vi "CREATE VECTOR FROM SELECTION.vi"(0 "RadioButtonsControl in":refnum<vi>, 1 "Ts (Sampling Rate)":u16(ring) items=["1000 sec"=0, "100 msec"=8, "10 msec"=4, "1 msec"=2, "100 usec"=1], 2 "Digital (pin2) conf":enum32{"Item 0", "Item 1"}(radio), 3 "A3":bool, 4 "Digital (pin4) conf":enum32{"Item 0", "Item 1"}(radio), 6 "RadioBtnsControl Refnum in":refnum<vi>, 7 "enable DIO":bool, 8 "A0":bool, 9 "A5":bool, 10 "A1":bool, 11 "A2":bool, 13 "A4":bool) -> (15 "Array":bool[](array[boolean]))   [LabVIEW 2018]
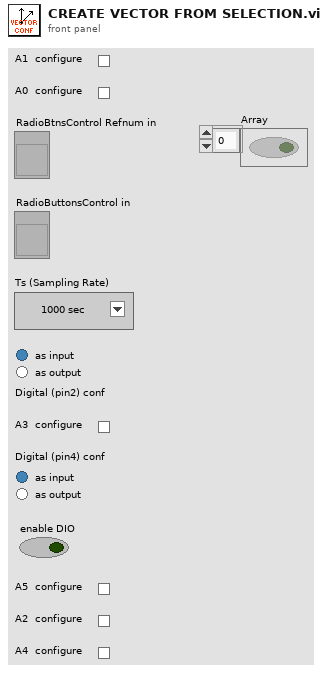
[diagram p1: front panel]
types:
  T1 = enum8{"Enabled", "Disabled", "Disabled and Grayed Out"}
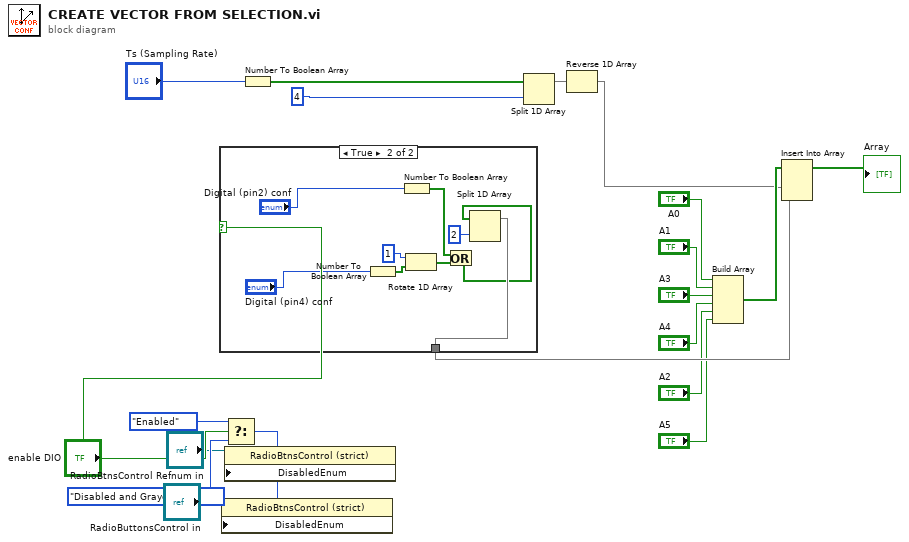
[diagram p0: block diagram]
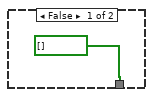
[diagram p2: hidden frame]
diagram:
  n1 = case shown="True" "enable DIO" {
    tunnel: [bool[] [] ("x .or. y?") w24] -> w19
    frame False {
    }
    frame True {
      n2 = Number To Boolean Array(number="Digital (pin4) conf") -> (Boolean array=w28:bool[])
      n3 = Number To Boolean Array(number="Digital (pin2) conf") -> (Boolean array=w29:bool[])
      n4 = Rotate 1D Array(1:w28, 2:1 ("n")) -> (0:w27:bool[])
      n5 = Or(x=w29, y=w27) -> (x .or. y?=w23:bool[])
      n6 = Split 1D Array(array=w23, index=2) -> (first subarray=w24:bool[])  [unwired: 1 out]
    }
  }
  n7 = Select(t=T1."Enabled" ("Disabled"), s="enable DIO", f=T1."Disabled and Grayed Out" ("Disabled")) -> (s? t:f=w16:T1)
  n8 = property on="Property Node" class="RadioBtnsControl (strict)"(reference="RadioButtonsControl in", "DisabledEnum"=w16) -> ()  [unwired: 1 in, 2 out]
  n9 = property on="Property Node" class="RadioBtnsControl (strict)"(reference="RadioBtnsControl Refnum in", "DisabledEnum"=w16) -> ()  [unwired: 1 in, 2 out]
  n10 = Number To Boolean Array(number="Ts (Sampling Rate)") -> (Boolean array=w10:bool[])
  n11 = Split 1D Array(array=w10, index=4) -> (first subarray=w12:bool[])  [unwired: 1 out]
  n12 = Reverse 1D Array(array=w12) -> (reversed array=w13:bool[])
  n13 = Build Array("A0", "A1", "A3", "A4", "A2", "A5") -> (w18:bool[])
  n14 = Insert Into Array(array=w18, new element #1=w13, new element #2=w19) -> (→"Array":bool[])  [unwired: 1 in]
